vi "Untitled 1.vi"() -> ()   [LabVIEW 2018]
uses:
  MICAS-X/Template Scripting/Driver Creator/Driver Creator.lvclass
panel:
  out "VI Refs out":refnum<vi>[](array[refnum])
  out "Driver Creator out":refnum<class "Driver Creator.lvclass">
  in  "Driver Creator in":refnum<class "Driver Creator.lvclass">
  out "error out":errorcluster
  in  "error in (no error)":errorcluster
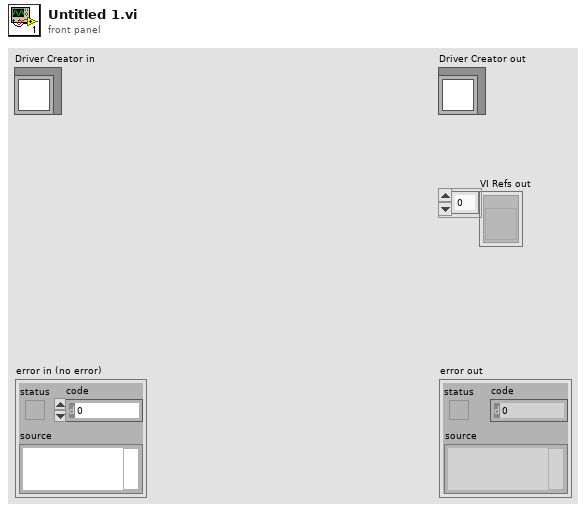
[diagram p1: front panel]
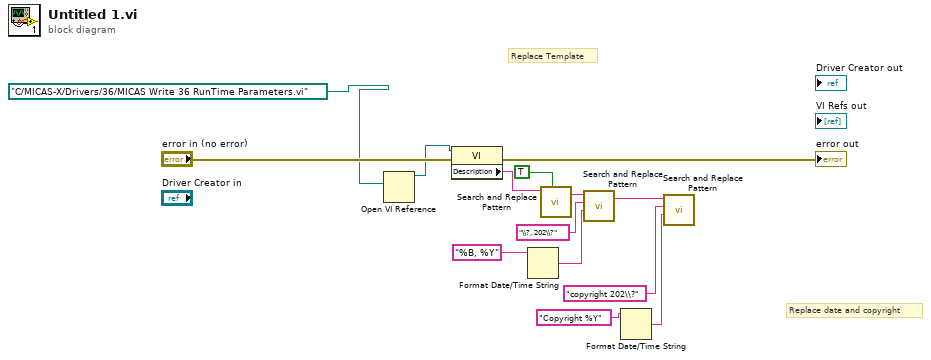
[diagram p0: block diagram]
diagram:
  # "Replace date and copyright"
  # "Replace Template"
  n1 = Open VI Reference(vi path=path "C:/MICAS-X/Drivers/36/MICAS Write 36 RunTime Parameters.vi") -> (vi reference=w1:refnum<vi>)  [unwired: 5 in, 1 out]
  n2 = property class="VI"(reference=w1, error in="error in (no error)") -> (error out=→"error out":errorcluster, "Description"=w11:string)  [unwired: 1 out]
  n3 = Format Date/Time String(time format string (%c)="%B, %Y") -> (date/time string=w5:string)  [unwired: 2 in]
  n4 = call <vilib>:"Search and Replace Pattern.vi"("string"=w11, "replace all? (F)"=TRUE) -> ("result string"=w9:string)  [unwired: 3 in, 1 out]
  n5 = call <vilib>:"Search and Replace Pattern.vi"("string"=w9, "regular expression (\"\")"="\\?, 202\\?", "replace string (\"\")"=w5) -> ("result string"=w8:string)  [unwired: 2 in, 1 out]
  n6 = Format Date/Time String(time format string (%c)="Copyright %Y") -> (date/time string=w3:string)  [unwired: 2 in]
  n7 = call <vilib>:"Search and Replace Pattern.vi"("string"=w8, "regular expression (\"\")"="copyright 202\\?" ("regular expression (\"\")"), "replace string (\"\")"=w3) -> ()  [unwired: 2 in, 2 out]
